vi "Get ILIM.vi"(8 "error in":errorcluster, 11 "SR 3XX HVPS in":refnum<class "SR 3XX HVPS.lvclass">) -> (0 "error out":errorcluster, 2 "ILIM":sgl, 3 "SR 3XX HVPS out":refnum<class "SR 3XX HVPS.lvclass">)   [LabVIEW 2014, in "SR 3XX HVPS.lvclass"]
doc: "The ILIM? query returns the current limit setting."
uses:
  SR 3XX HVPS.lvclass
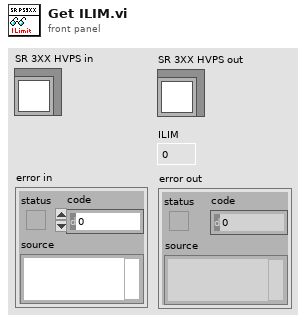
[diagram p1: front panel]
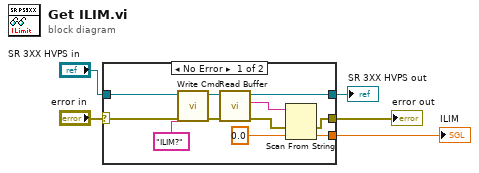
[diagram p0: block diagram]
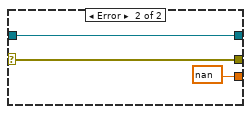
[diagram p2: hidden frame]
diagram:
  n1 = case shown="No Error" "error in" {
    selector: "error in" -> [w12 w19]
    tunnel: [w8 w19] -> w4
    tunnel: [w11 w18] -> w2
    tunnel: "SR 3XX HVPS in" -> [w16 w18]
    tunnel: [w6 sgl nan] -> w1
    frame No Error {
      n2 = call "Write Cmd.vi"("error in"=w12, "Cmd"="ILIM?", "SR 3XX HVPS in"=w16) -> ("error out"=w13:errorcluster, "SR 3XX HVPS out"=w14:refnum<class "SR 3XX HVPS.lvclass">)  [unwired: 7 in]
      n3 = call "Read Buffer.vi"("error in"=w13, "SR 3XX HVPS in"=w14) -> ("error out"=w9:errorcluster, "ReadData"=w10:string, "SR 3XX HVPS out"=w11:refnum<class "SR 3XX HVPS.lvclass">)  [unwired: 7 in]
      n4 = Scan From String(input string=w10, error in=w9, default 1=sgl 0.0 ("default (0 dbl)")) -> (error out=w8:errorcluster, output 1=w6:sgl)  [unwired: 2 in, 2 out]
    }
    frame Error {
    }
  }
  "error out" <- w4
  "SR 3XX HVPS out" <- w2
  "ILIM" <- w1
